vi "TestZscan.vi"() -> ()   [LabVIEW 2018]
uses:
  <vilib>/Instr/_visa.llb/VISA Configure Serial Port (Instr).vi
panel:
  out "error out":errorcluster
  out "read buffer":string
  in  "stop":bool
  in  "VISA resource name":refnum<visa-resource-name>
  out "error out 2":errorcluster
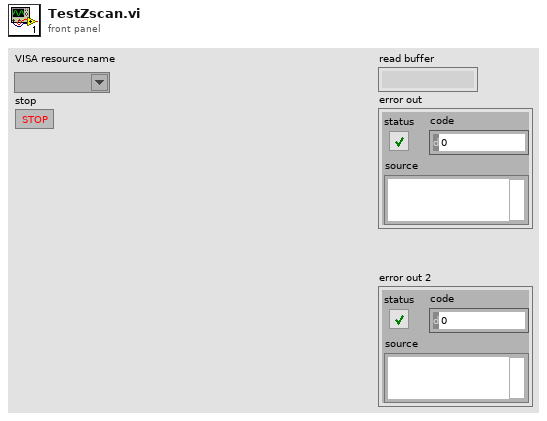
[diagram p1: front panel]
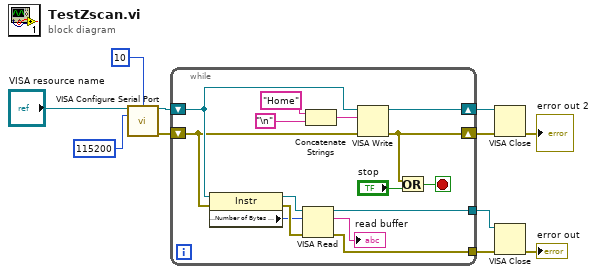
[diagram p0: block diagram]
diagram:
  n1 = call-poly "VISA Configure Serial Port"("VISA resource name"="VISA resource name", "termination char\n(0xA = '\\n' = LF)"=u8 10 ("termination char\n(0xA = '\\n' = LF)"), "baud rate (9600)"=u32 115200) -> ("VISA resource name out"=w4:refnum<visa-resource-name>, "error out"=w3:errorcluster)  [unwired: 11 in]
  n2 = while {
    tunnel: [w18] -> w6
    tunnel: [w17] -> w5
    shift-right: [w26] -> w10
    shift-left: w4 -> [w15]
    shift-right: [w25] -> w9
    shift-left: w3 -> [w14]
    stop <- w12 stop-if-true
    n3 = property class="Instr"(reference=w15, error in=w14) -> (reference out=w20:refnum<visa-resource-name>, error out=w19:errorcluster, "Serial Settings:Number of Bytes at Serial Port"=w16:u32)
    n4 = VISA Read(VISA resource name=w20, byte count=w16, error in (no error)=w19) -> (VISA resource name out=w18:refnum<visa-resource-name>, read buffer=→"read buffer":string, error out=w17:errorcluster)  [unwired: 1 out]
    n5 = Concatenate Strings("Home", "\n") -> (w21:string)
    n6 = VISA Write(VISA resource name=w15, write buffer=w21, error in (no error)=w14) -> (VISA resource name out=w26:refnum<visa-resource-name>, error out=w25:errorcluster)  [unwired: 1 out]
    n7 = Or(x=w25, y="stop") -> (x .or. y?=w12:bool)
  }
  n8 = VISA Close(VISA resource name=w10, error in (no error)=w9) -> (error out=→"error out 2":errorcluster)
  n9 = VISA Close(VISA resource name=w6, error in (no error)=w5) -> (error out=→"error out":errorcluster)
